vi "CAlex2_Display_NoCables.vi"(4 "AnkleTraj":dbl[][](array[numeric]), 5 "ClosePt":dbl[](array[numeric]), 6 "Init?":bool, 8 "error in (no error)":errorcluster, 9 "AxisSetting":T1={"AxisLabel"=["x ", "y", "z "], "AxisMax"=[0.6, 0.7, 0.2], "AxisMin"=[-0.4, -0.3, -0.8]}, 10 "3D graph in":refnum<k7>, 11 "CLX2 in":refnum<class "CAlex2_Display.lvclass">) -> (0 "error out":errorcluster, 1 "LastPlotNum":i32=1, 2 "3D graph out":refnum<k7>, 3 "CLX2 out":refnum<class "CAlex2_Display.lvclass">)   [LabVIEW 2015, in "CAlex2_Display.lvclass"]
uses:
  CAlex2_Display.lvclass
  <vilib>/Platform/NI_3dgraph.lvlib
  <vilib>/ptbypt/NI_PtbyPt.lvlib
  SerialChain-Cable/SerialChain-Cable.lvclass
panel:
  out "EndEffInGCS":dbl[](array[numeric]) format="%#.6f"
  in  "sample length":i32=15
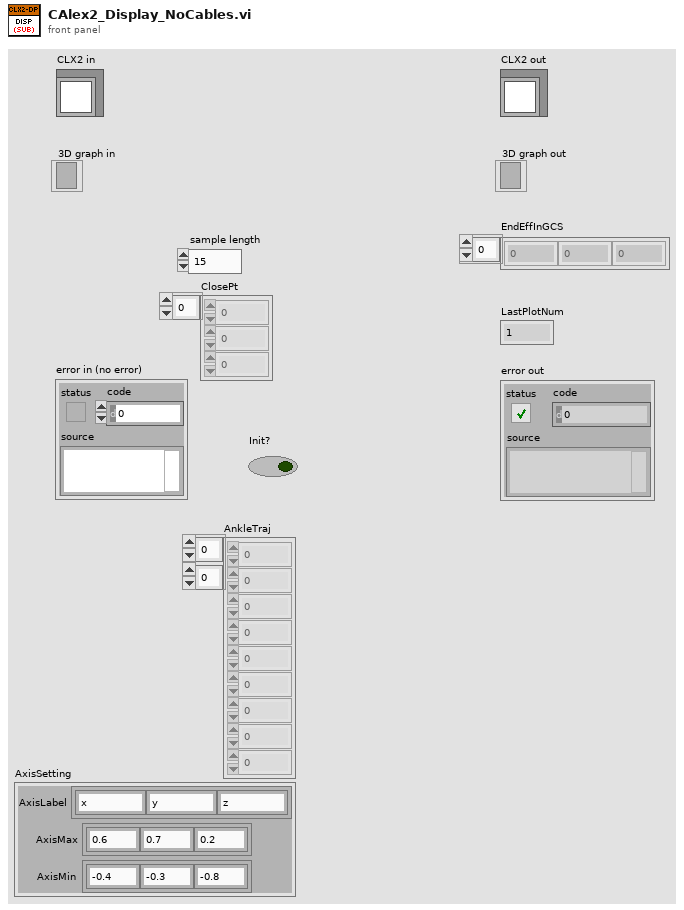
[diagram p1: front panel]
types:
  T1 = cluster{"AxisLabel":string[], "AxisMax":dbl[], "AxisMin":dbl[]}
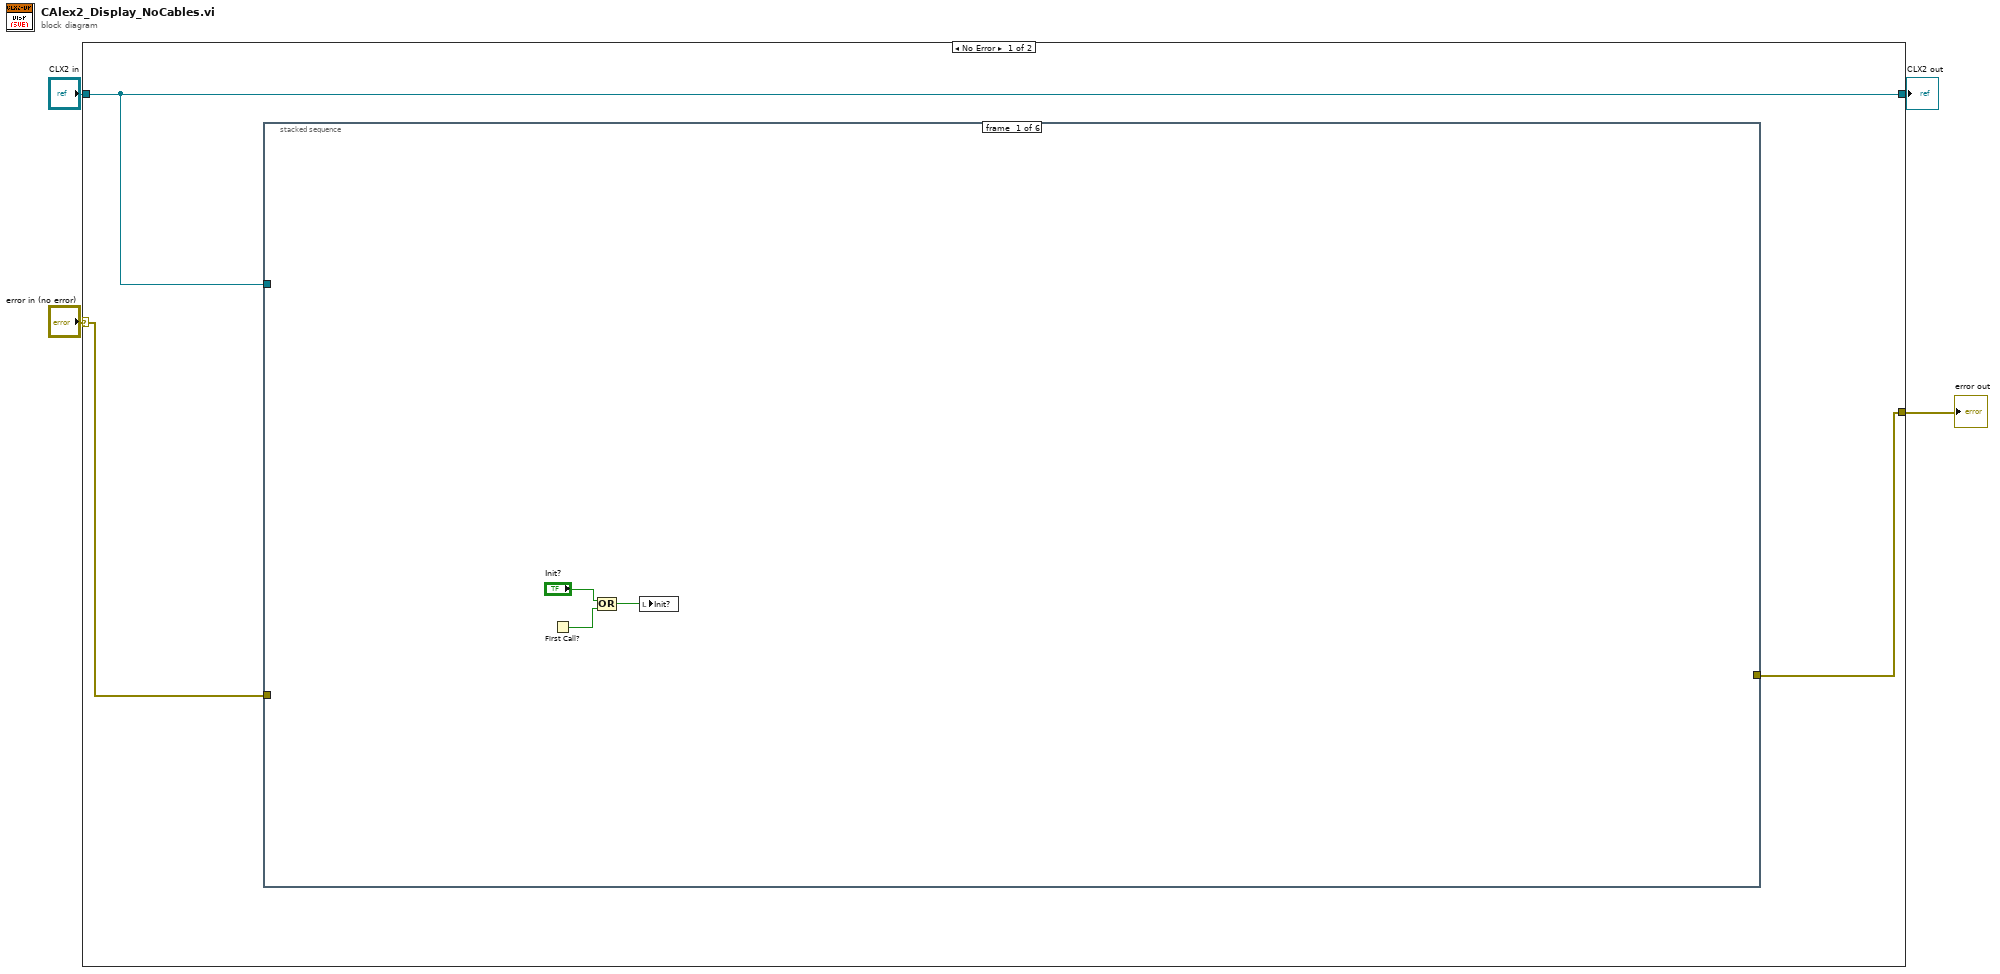
[diagram p0: block diagram]
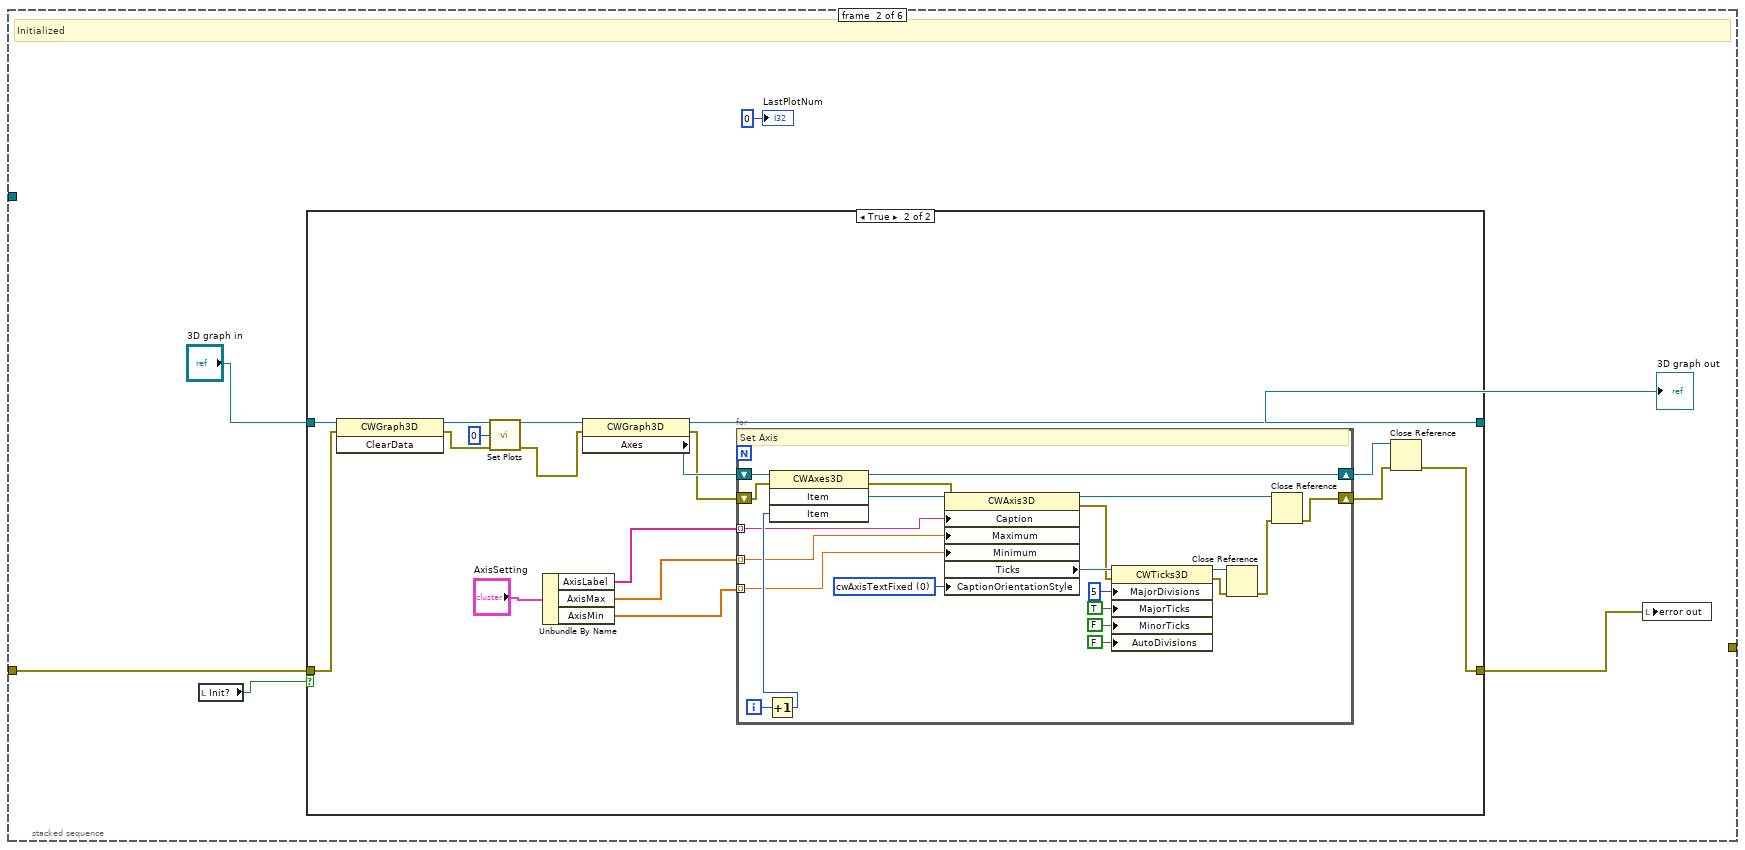
[diagram p2: hidden frame]
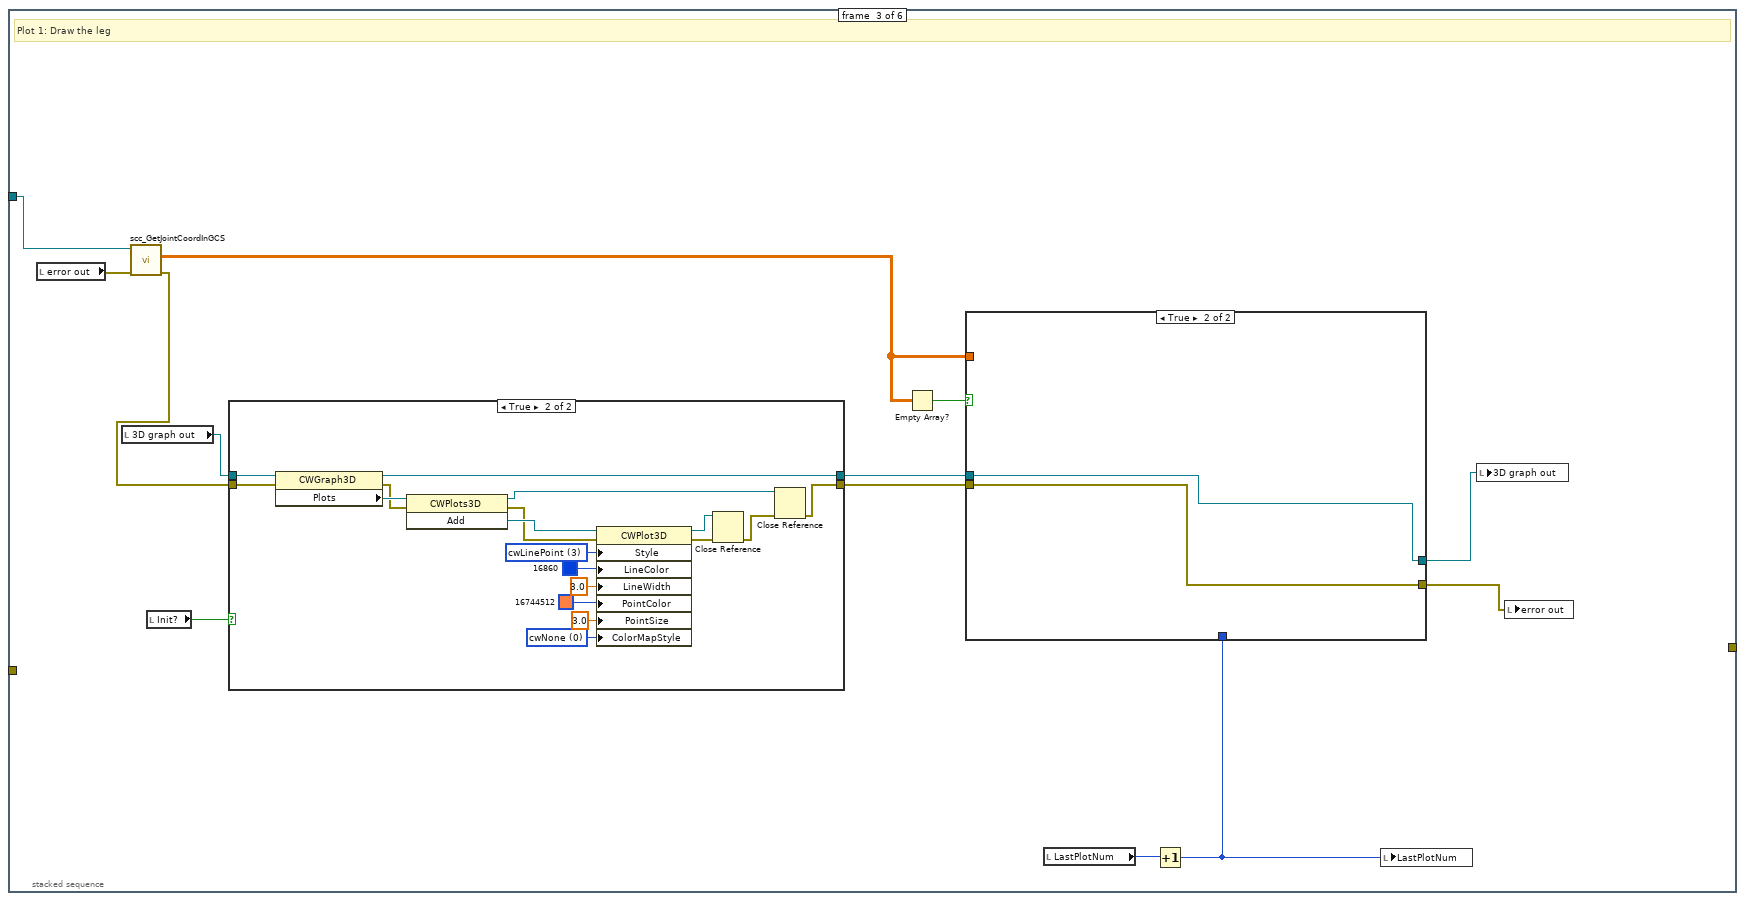
[diagram p4: hidden frame]
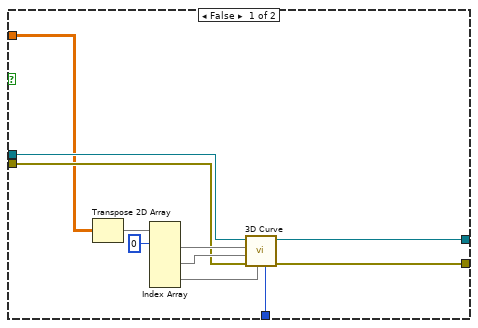
[diagram p5: hidden frame]
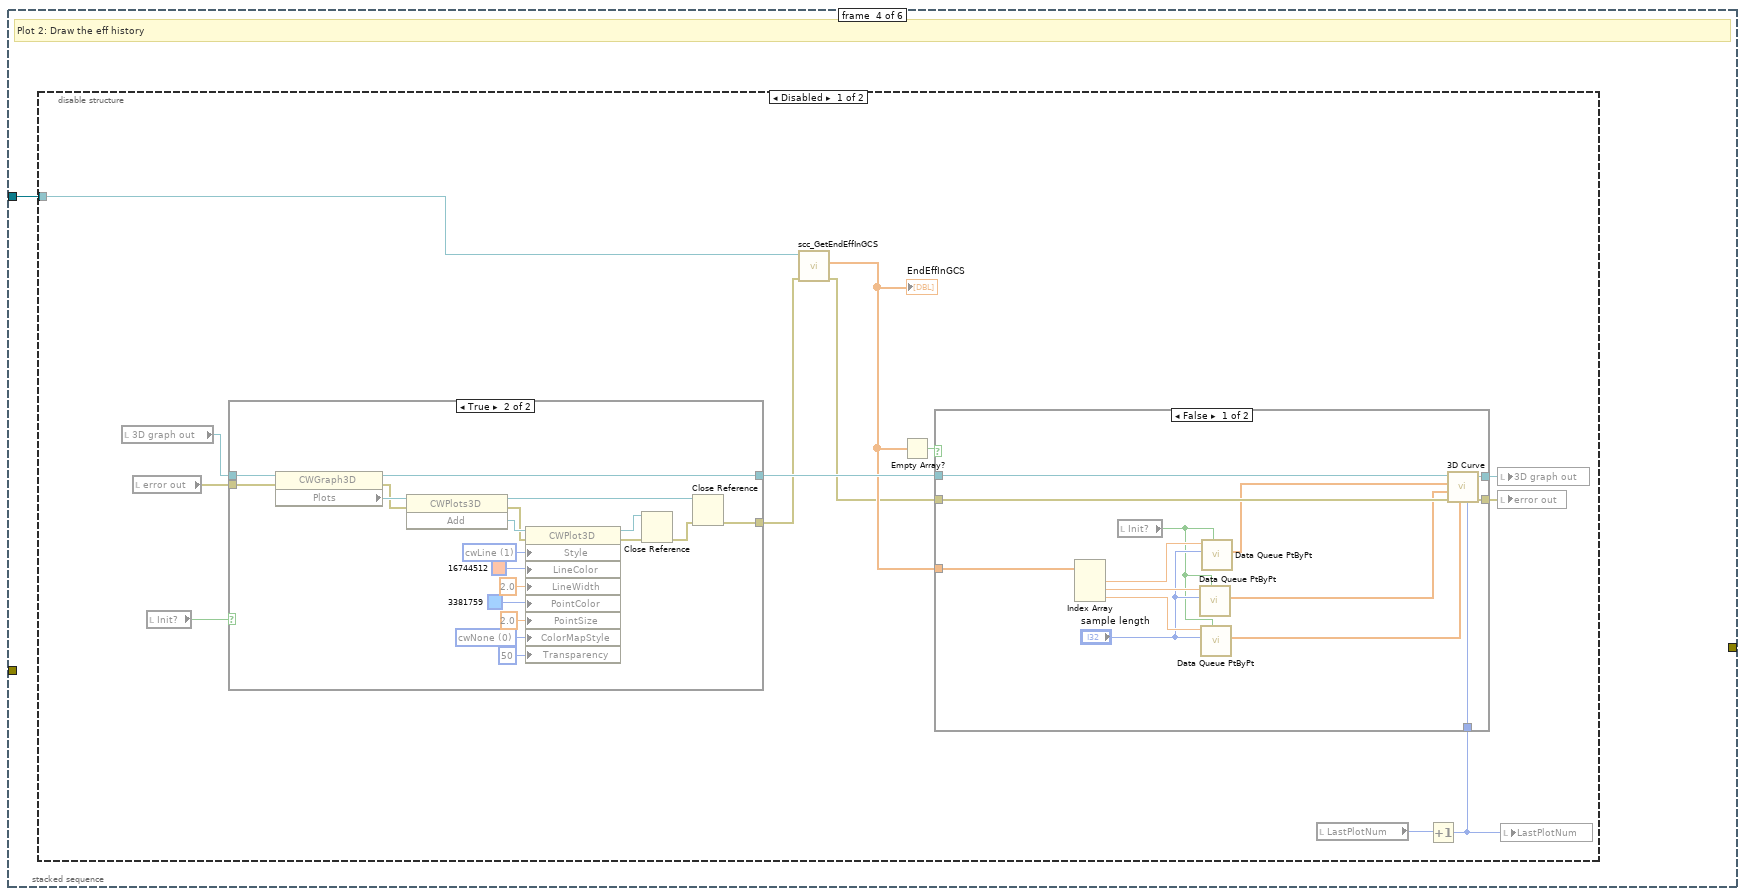
[diagram p7: hidden frame]
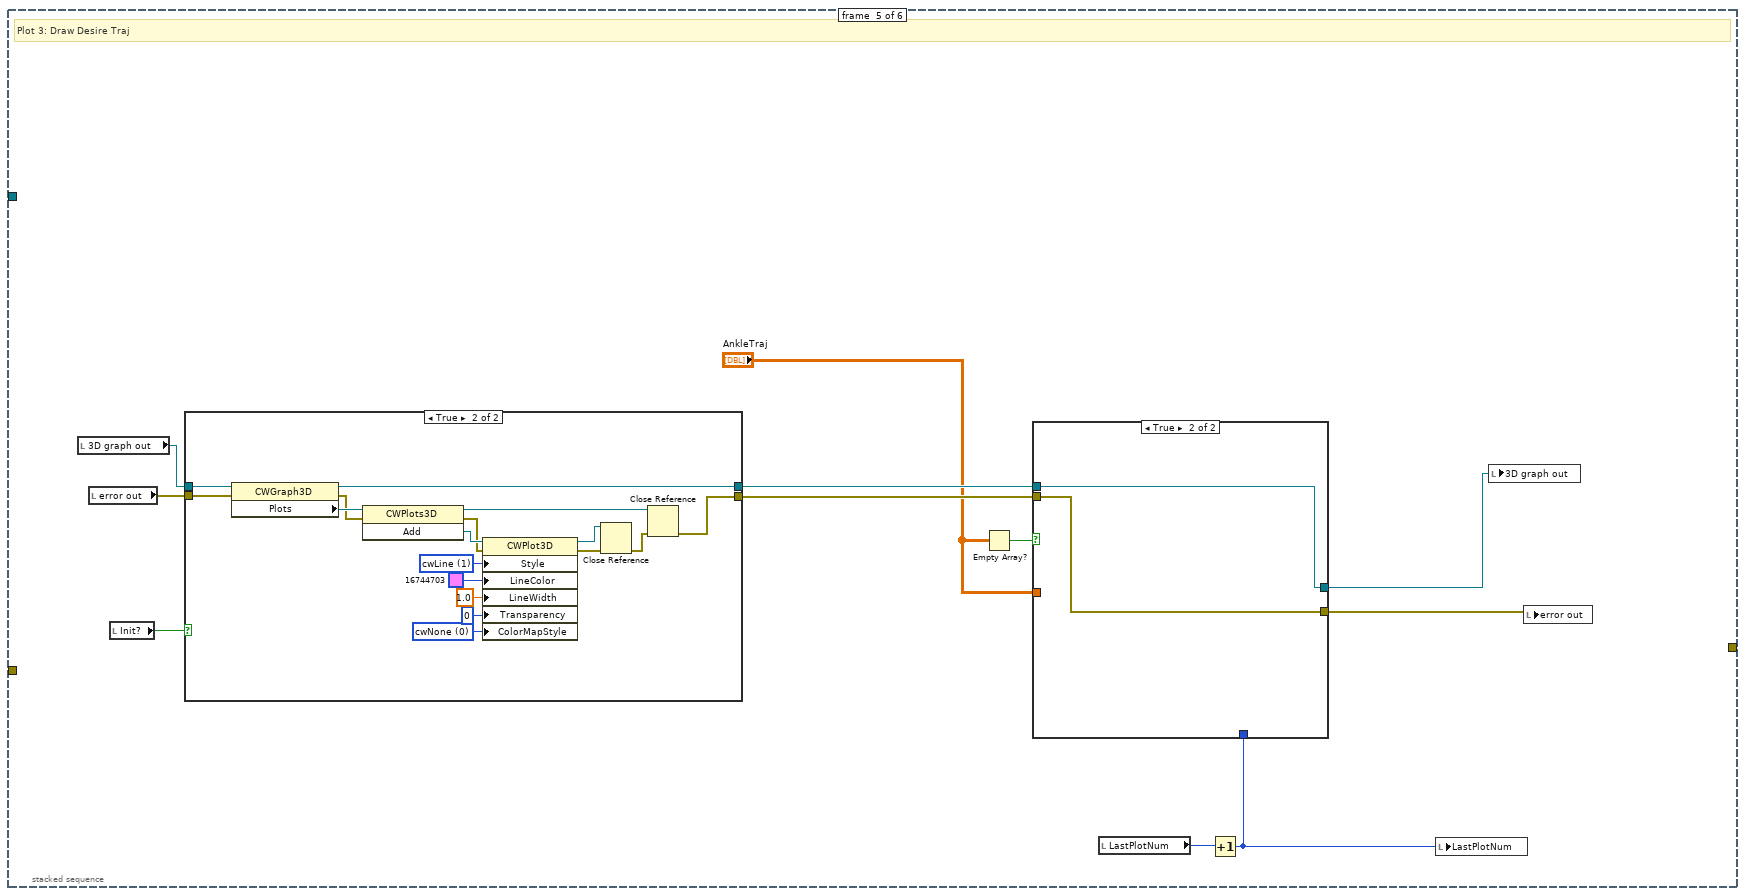
[diagram p11: hidden frame]
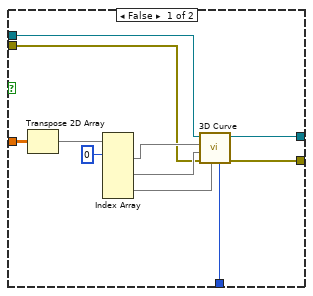
[diagram p12: hidden frame]
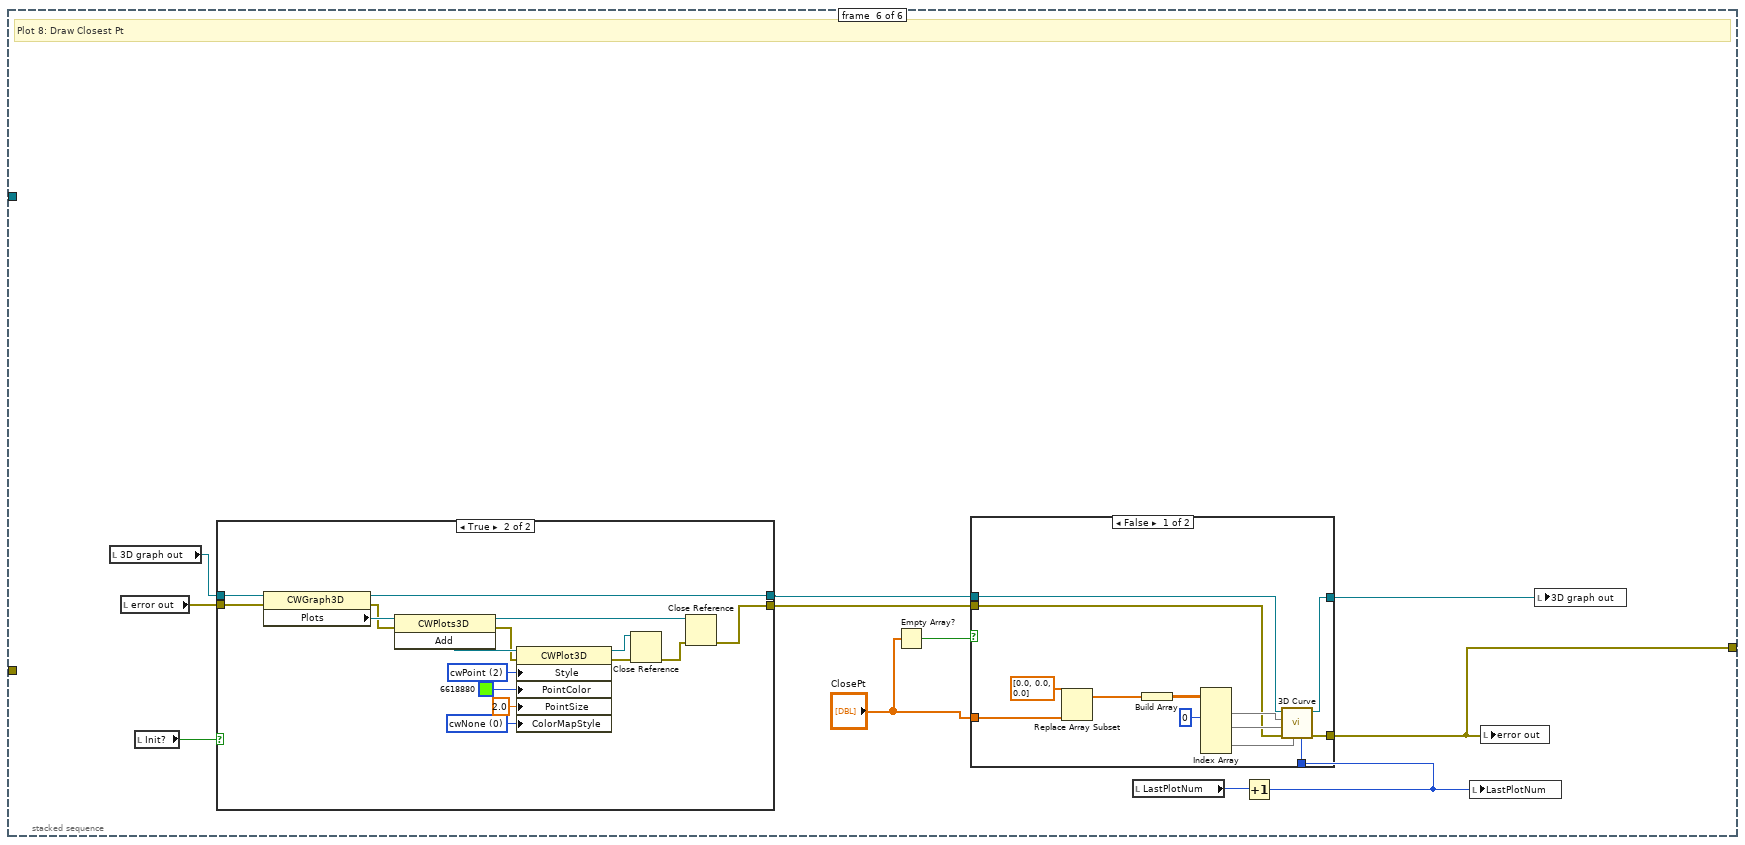
[diagram p14: hidden frame]
diagram:
  n1 = case shown="No Error" "error in (no error)" {
    selector: "error in (no error)" -> [w6 w243]
    tunnel: [w7 w243] -> w1
    tunnel: [w5 w242] -> w2
    tunnel: "CLX2 in" -> [w5 w242]
    frame No Error {
      n2 = stacked-sequence {
        tunnel: [_ _ _ _ _ w198] -> w7
        tunnel: w6 -> [_ w12 _ _ _ _]
        tunnel: w5 -> [_ _ w68 w104 _ _]
        frame #0 {
          n3 = First Call?() -> (First Call?: T/F=w10:bool)
          n4 = Or(x="Init?", y=w10) -> (x .or. y?=w8:bool)
          n5 = local write "Init?"(w8) -> ()
        }
        frame #1 {
          # "Initialized"
          n6 = local read "Init?"() -> (w11:bool)
          n7 = case shown="True" w11 {
            tunnel: "3D graph in" -> [w18 w32]
            tunnel: [w18 w28] -> w15
            tunnel: [w17 w23] -> w13
            tunnel: w12 -> [w17 w30]
            frame False {
            }
            frame True {
              n8 = invoke class="CWGraph3D" method="ClearData"(reference=w32, error in=w30) -> (reference out=w31:refnum<k7>, error out=w29:errorcluster)  [unwired: 1 in, 1 out]
              n9 = call <vilib>:"Set Plots.vi"("3D graph"=w31, "# of plots(1)"=0, "error in (no error)"=w29) -> ("3D graph out"=w33:refnum<k7>, "error out"=w24:errorcluster)  [unwired: 11 in]
              n10 = Unbundle By Name("AxisSetting") -> ("AxisLabel"=w21:string[], "AxisMax"=w20:dbl[], "AxisMin"=w19:dbl[])
              n11 = property class="CWGraph3D"(reference=w33, error in=w24) -> (reference out=w28:refnum<k7>, error out=w25:errorcluster, "Axes"=w34:refnum<k7>)
              n12 = for {
                shift-right: [w44] -> w26
                shift-left: w34 -> [w57]
                shift-right: [w45] -> w27
                shift-left: w25 -> [w42]
                tunnel: w21 -> [w38] mode=indexing
                tunnel: w20 -> [w37] mode=indexing
                tunnel: w19 -> [w36] mode=indexing
                i -> [w40]
                w41 = 0 items=["cwAxisTextFixed", "cwAxisTextFaceCamera"] ("CaptionOrientationStyle")
                # "Set Axis"
                n13 = Increment(x=w40) -> (x+1=w39:i32)
                n14 = invoke class="CWAxes3D" method="Item"(reference=w57, error in=w42, "Item"=w39) -> (reference out=w44:refnum<k7>, error out=w43:errorcluster, "Item"=w56:refnum<k7>)  [unwired: 1 in, 1 out]
                n15 = property class="CWAxis3D"(reference=w56, error in=w43, "Caption"=w38, "Maximum"=w37, "Minimum"=w36, "CaptionOrientationStyle"=w41) -> (reference out=w46:refnum<k7>, error out=w49:errorcluster, "Ticks"=w55:refnum<k7>)
                n16 = property class="CWTicks3D"(reference=w55, error in=w49, "MajorDivisions"=5, "MajorTicks"=TRUE, "MinorTicks"=FALSE, "AutoDivisions"=FALSE) -> (reference out=w48:refnum<k7>, error out=w50:errorcluster)
                n17 = Close Reference(reference=w48, error in (no error)=w50) -> (error out=w47:errorcluster)
                n18 = Close Reference(reference=w46, error in (no error)=w47) -> (error out=w45:errorcluster)
              }
              n19 = Close Reference(reference=w26, error in (no error)=w27) -> (error out=w23:errorcluster)
            }
          }
          "3D graph out" <- w15
          n20 = local write "error out"(w13) -> ()
          "LastPlotNum" <- 0 ("LastPlotNum 2")
        }
        frame #2 {
          # "Plot 1: Draw the leg"
          n21 = local read "error out"() -> (w60:errorcluster)
          n22 = local read "3D graph out"() -> (w66:refnum<k7>)
          n23 = call "scc_GetJointCoordInGCS.vi"("error in (no error)"=w60, "SerialChain_Cable in"=w68) -> ("error out"=w59:errorcluster, "Joint Coord in GCS"=w58:dbl[][])  [unwired: 5 in, 3 out]
          n24 = local read "Init?"() -> (w62:bool)
          n25 = case shown="True" w62 {
            tunnel: w59 -> [w84 w97]
            tunnel: w66 -> [w85 w92]
            tunnel: [w85 w91] -> w65
            tunnel: [w84 w86] -> w64
            frame False {
            }
            frame True {
              w90 = 0 items=["cwNone", "cwShaded", "cwColorSpectrum", "cwGrayScale", "cwCustom"] ("ColorMapStyle")
              w103 = 3 items=["cwLine"=1, "cwPoint"=2, "cwLinePoint"=3, "cwHiddenLine"=4, "cwSurface"=5, "cwSurfaceLine"=6, "cwSurfaceNormal"=7, "cwContourLine"=8, "cwSurfaceContour"=9] ("Style")
              n26 = property class="CWGraph3D"(reference=w92, error in=w97) -> (reference out=w91:refnum<k7>, error out=w100:errorcluster, "Plots"=w101:refnum<k7>)
              n27 = invoke class="CWPlots3D" method="Add"(reference=w101, error in=w100) -> (reference out=w88:refnum<k7>, error out=w89:errorcluster, "Add"=w102:refnum<k7>)  [unwired: 1 in]
              n28 = property class="CWPlot3D"(reference=w102, error in=w89, "Style"=w103, "LineColor"=u32 16860, "LineWidth"=3.0, "PointColor"=u32 16744512, "PointSize"=3.0 ("LineWidth"), "ColorMapStyle"=w90) -> (reference out=w98:refnum<k7>, error out=w99:errorcluster)
              n29 = Close Reference(reference=w98, error in (no error)=w99) -> (error out=w87:errorcluster)
              n30 = Close Reference(reference=w88, error in (no error)=w87) -> (error out=w86:errorcluster)
            }
          }
          n31 = Empty Array?(array=w58) -> (empty?=w61:bool)
          n32 = local read "LastPlotNum"() -> (w70:i32)
          n33 = Increment(x=w70) -> (x+1=w69:i32)
          n34 = case shown="True" w61 {
            tunnel: [w76 w83] -> w67
            tunnel: w65 -> [w75 w83]
            tunnel: w64 -> [w74 w82]
            tunnel: [w73 w82] -> w63
            tunnel: w69 -> [w72 _]
            tunnel: w58 -> [w71 _]
            frame False {
              n35 = Transpose 2D Array(2D array=w71) -> (transposed array=w77:dbl[][])
              n36 = Index Array(array=w77, index (row) #1=0 ("index (row)")) -> (element #1=w79:dbl[], element #2=w80:dbl[], element #3=w81:dbl[])  [unwired: 5 in]
              n37 = call <vilib>:"3D Curve.vi"("plot number (1)"=w72, "z vector"=w81, "error in (no error)"=w74, "y vector"=w80, "x vector"=w79, "3D graph"=w75) -> ("error out"=w73:errorcluster, "3D graph out"=w76:refnum<k7>)  [unwired: 4 in]
            }
            frame True {
            }
          }
          n38 = local write "LastPlotNum"(w69) -> ()
          n39 = local write "3D graph out"(w67) -> ()
          n40 = local write "error out"(w63) -> ()
        }
        frame #3 {
          # "Plot 2: Draw the eff history"
          n41 = disable-structure shown="Disabled" {
            disable-tunnel: w104 -> [w117 _]
            frame Disabled {
              n42 = local read "3D graph out"() -> (w112:refnum<k7>)
              n43 = local read "error out"() -> (w113:errorcluster)
              n44 = local read "Init?"() -> (w109:bool)
              n45 = case shown="True" w109 {
                tunnel: w113 -> [w134 w147]
                tunnel: w112 -> [w135 w142]
                tunnel: [w135 w141] -> w111
                tunnel: [w134 w136] -> w106
                frame False {
                }
                frame True {
                  w140 = 0 items=["cwNone", "cwShaded", "cwColorSpectrum", "cwGrayScale", "cwCustom"] ("ColorMapStyle")
                  w154 = 1 items=["cwLine"=1, "cwPoint"=2, "cwLinePoint"=3, "cwHiddenLine"=4, "cwSurface"=5, "cwSurfaceLine"=6, "cwSurfaceNormal"=7, "cwContourLine"=8, "cwSurfaceContour"=9] ("Style")
                  n46 = property class="CWGraph3D"(reference=w142, error in=w147) -> (reference out=w141:refnum<k7>, error out=w151:errorcluster, "Plots"=w152:refnum<k7>)
                  n47 = invoke class="CWPlots3D" method="Add"(reference=w152, error in=w151) -> (reference out=w150:refnum<k7>, error out=w138:errorcluster, "Add"=w153:refnum<k7>)  [unwired: 1 in]
                  n48 = property class="CWPlot3D"(reference=w153, error in=w138, "Style"=w154, "LineColor"=u32 16744512, "LineWidth"=2.0, "PointColor"=u32 3381759, "PointSize"=2.0 ("LineWidth"), "ColorMapStyle"=w140, "Transparency"=50) -> (reference out=w148:refnum<k7>, error out=w149:errorcluster)
                  n49 = Close Reference(reference=w148, error in (no error)=w149) -> (error out=w137:errorcluster)
                  n50 = Close Reference(reference=w150, error in (no error)=w137) -> (error out=w136:errorcluster)
                }
              }
              n51 = call "scc_GetEndEffInGCS.vi"("error in (no error)"=w106, "SerialChain_Cable in"=w117) -> ("error out"=w105:errorcluster, "Pendeff(GCS)"=w107:dbl[])  [unwired: 5 in, 3 out]
              "EndEffInGCS" <- w107
              n52 = Empty Array?(array=w107) -> (empty?=w108:bool)
              n53 = local read "LastPlotNum"() -> (w115:i32)
              n54 = Increment(x=w115) -> (x+1=w116:i32)
              n55 = case shown="False" w108 {
                tunnel: [w131 w133] -> w114
                tunnel: w111 -> [w130 w133]
                tunnel: w105 -> [w129 w132]
                tunnel: [w128 w132] -> w110
                tunnel: w116 -> [w127 _]
                tunnel: w107 -> [w118 _]
                frame False {
                  n56 = Index Array(array=w118) -> (element #1=w124:dbl, element #2=w125:dbl, element #3=w126:dbl)  [unwired: 3 in]
                  n57 = local read "Init?"() -> (w119:bool)
                  n58 = call <vilib>:"Data Queue PtByPt.vi"("initialize"=w119, "sample length"="sample length", "input data point"=w125) -> ("Current Queue"=w121:dbl[])  [unwired: 4 in, 4 out]
                  n59 = call <vilib>:"Data Queue PtByPt.vi"("initialize"=w119, "sample length"="sample length", "input data point"=w126) -> ("Current Queue"=w120:dbl[])  [unwired: 4 in, 4 out]
                  n60 = call <vilib>:"Data Queue PtByPt.vi"("initialize"=w119, "sample length"="sample length", "input data point"=w124) -> ("Current Queue"=w122:dbl[])  [unwired: 4 in, 4 out]
                  n61 = call <vilib>:"3D Curve.vi"("plot number (1)"=w127, "z vector"=w120, "error in (no error)"=w129, "y vector"=w121, "x vector"=w122, "3D graph"=w130) -> ("error out"=w128:errorcluster, "3D graph out"=w131:refnum<k7>)  [unwired: 4 in]
                }
                frame True {
                }
              }
              n62 = local write "3D graph out"(w114) -> ()
              n63 = local write "error out"(w110) -> ()
              n64 = local write "LastPlotNum"(w116) -> ()
            }
            frame Enabled {
            }
          }
        }
        frame #4 {
          # "Plot 3: Draw Desire Traj"
          n65 = local read "3D graph out"() -> (w161:refnum<k7>)
          n66 = local read "error out"() -> (w162:errorcluster)
          n67 = local read "Init?"() -> (w159:bool)
          n68 = case shown="True" w159 {
            tunnel: w162 -> [w179 w190]
            tunnel: w161 -> [w180 w187]
            tunnel: [w180 w186] -> w160
            tunnel: [w179 w181] -> w158
            frame False {
            }
            frame True {
              w184 = 0 items=["cwNone", "cwShaded", "cwColorSpectrum", "cwGrayScale", "cwCustom"] ("ColorMapStyle")
              w197 = 1 items=["cwLine"=1, "cwPoint"=2, "cwLinePoint"=3, "cwHiddenLine"=4, "cwSurface"=5, "cwSurfaceLine"=6, "cwSurfaceNormal"=7, "cwContourLine"=8, "cwSurfaceContour"=9] ("Style")
              n69 = property class="CWGraph3D"(reference=w187, error in=w190) -> (reference out=w186:refnum<k7>, error out=w194:errorcluster, "Plots"=w195:refnum<k7>)
              n70 = invoke class="CWPlots3D" method="Add"(reference=w195, error in=w194) -> (reference out=w193:refnum<k7>, error out=w183:errorcluster, "Add"=w196:refnum<k7>)  [unwired: 1 in]
              n71 = property class="CWPlot3D"(reference=w196, error in=w183, "Style"=w197, "LineColor"=u32 16744703, "LineWidth"=1.0, "Transparency"=0, "ColorMapStyle"=w184) -> (reference out=w191:refnum<k7>, error out=w192:errorcluster)
              n72 = Close Reference(reference=w191, error in (no error)=w192) -> (error out=w182:errorcluster)
              n73 = Close Reference(reference=w193, error in (no error)=w182) -> (error out=w181:errorcluster)
            }
          }
          n74 = Empty Array?(array="AnkleTraj") -> (empty?=w156:bool)
          n75 = local read "LastPlotNum"() -> (w165:i32)
          n76 = Increment(x=w165) -> (x+1=w164:i32)
          n77 = case shown="True" w156 {
            tunnel: "AnkleTraj" -> [w176 _]
            tunnel: [w170 w178] -> w163
            tunnel: w160 -> [w169 w178]
            tunnel: w164 -> [w168 _]
            tunnel: w158 -> [w167 w177]
            tunnel: [w166 w177] -> w157
            frame False {
              n78 = Transpose 2D Array(2D array=w176) -> (transposed array=w171:dbl[][])
              n79 = Index Array(array=w171, index (row) #1=0 ("index (row)")) -> (element #1=w173:dbl[], element #2=w174:dbl[], element #3=w175:dbl[])  [unwired: 5 in]
              n80 = call <vilib>:"3D Curve.vi"("plot number (1)"=w168, "z vector"=w175, "error in (no error)"=w167, "y vector"=w174, "x vector"=w173, "3D graph"=w169) -> ("error out"=w166:errorcluster, "3D graph out"=w170:refnum<k7>)  [unwired: 4 in]
            }
            frame True {
            }
          }
          n81 = local write "LastPlotNum"(w164) -> ()
          n82 = local write "3D graph out"(w163) -> ()
          n83 = local write "error out"(w157) -> ()
        }
        frame #5 {
          # "Plot 8: Draw Closest Pt"
          n84 = local read "3D graph out"() -> (w206:refnum<k7>)
          n85 = local read "error out"() -> (w207:errorcluster)
          n86 = local read "Init?"() -> (w205:bool)
          n87 = case shown="True" w205 {
            tunnel: w207 -> [w224 w234]
            tunnel: w206 -> [w225 w231]
            tunnel: [w225 w230] -> w204
            tunnel: [w224 w226] -> w201
            frame False {
            }
            frame True {
              w229 = 0 items=["cwNone", "cwShaded", "cwColorSpectrum", "cwGrayScale", "cwCustom"] ("ColorMapStyle")
              w241 = 2 items=["cwLine"=1, "cwPoint"=2, "cwLinePoint"=3, "cwHiddenLine"=4, "cwSurface"=5, "cwSurfaceLine"=6, "cwSurfaceNormal"=7, "cwContourLine"=8, "cwSurfaceContour"=9] ("Style")
              n88 = property class="CWGraph3D"(reference=w231, error in=w234) -> (reference out=w230:refnum<k7>, error out=w238:errorcluster, "Plots"=w239:refnum<k7>)
              n89 = invoke class="CWPlots3D" method="Add"(reference=w239, error in=w238) -> (reference out=w237:refnum<k7>, error out=w228:errorcluster, "Add"=w240:refnum<k7>)  [unwired: 1 in]
              n90 = property class="CWPlot3D"(reference=w240, error in=w228, "Style"=w241, "PointColor"=u32 6618880, "PointSize"=2.0 ("LineWidth"), "ColorMapStyle"=w229) -> (reference out=w235:refnum<k7>, error out=w236:errorcluster)
              n91 = Close Reference(reference=w235, error in (no error)=w236) -> (error out=w227:errorcluster)
              n92 = Close Reference(reference=w237, error in (no error)=w227) -> (error out=w226:errorcluster)
            }
          }
          n93 = Empty Array?(array="ClosePt") -> (empty?=w199:bool)
          n94 = local read "LastPlotNum"() -> (w203:i32)
          n95 = Increment(x=w203) -> (x+1=w202:i32)
          n96 = case shown="False" w199 {
            tunnel: "ClosePt" -> [w220 _]
            tunnel: [w213 w223] -> w208
            tunnel: w204 -> [w212 w223]
            tunnel: w202 -> [w211 _]
            tunnel: w201 -> [w210 w222]
            tunnel: [w209 w222] -> w198
            frame False {
              n97 = Replace Array Subset(array=dbl[] [0.0, 0.0, 0.0], new element=w220) -> (w219:dbl[])  [unwired: 1 in]
              n98 = Build Array(w219) -> (w218:dbl[][])
              n99 = Index Array(array=w218, index (col) #1=0 ("disabled index (col)")) -> (element #1=w216:dbl[], element #2=w215:dbl[], element #3=w214:dbl[])  [unwired: 5 in]
              n100 = call <vilib>:"3D Curve.vi"("plot number (1)"=w211, "z vector"=w214, "error in (no error)"=w210, "y vector"=w215, "x vector"=w216, "3D graph"=w212) -> ("error out"=w209:errorcluster, "3D graph out"=w213:refnum<k7>)  [unwired: 4 in]
            }
            frame True {
            }
          }
          n101 = local write "LastPlotNum"(w202) -> ()
          n102 = local write "error out"(w198) -> ()
          n103 = local write "3D graph out"(w208) -> ()
        }
      }
    }
    frame Error {
    }
  }
  "CLX2 out" <- w2
  "error out" <- w1
